vi "Memory.Pointer.Object To Block Descriptor.vi"(8 "error in (no error)":errorcluster, 11 "pointer in":refnum<class "Memory.Pointer.lvclass">) -> (0 "error out":errorcluster, 2 "block descriptor":cluster{"address":u64, "size":u64} {"address" format="%016x"; "size" format="%d bytes"}, 3 "pointer out":refnum<class "Memory.Pointer.lvclass">)   [LabVIEW 2016, in "Memory Manager.lvlib" / "Memory.Pointer.lvclass"]
uses:
  Memory.Pointer.lvclass
  Memory.Pointer.lvclass/Memory.Pointer.ctl
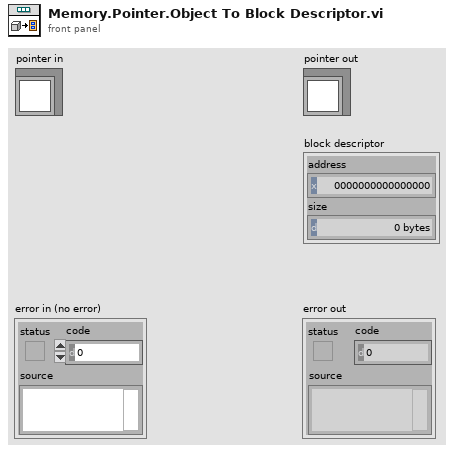
[diagram p1: front panel]
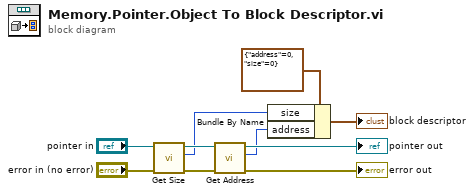
[diagram p0: block diagram]
diagram:
  n1 = call "Get Size.vi"("error in (no error)"="error in (no error)", "Pointer in"="pointer in") -> ("error out"=w8:errorcluster, "size"=w4:u64, "Pointer out"=w9:refnum<class "Memory.Pointer.lvclass">)  [unwired: 7 in]
  n2 = call "Get Address.vi"("error in (no error)"=w8, "Pointer in"=w9) -> ("error out"=→"error out":errorcluster, "address"=w1:u64, "Pointer out"=→"pointer out":refnum<class "Memory.Pointer.lvclass">)  [unwired: 7 in]
  n3 = Bundle By Name(cluster=cluster{"address":u64, "size":u64} {"address"=0, "size"=0} ("input cluster"), "size"=w4, "address"=w1) -> (→"block descriptor":cluster{"address":u64, "size":u64})
